vi "Create Phrase with Unit or Greek Letter.vi"(0 "Phrase IN":refnum<k24>, 2 "Exponent rise":sgl, 5 "Greek Font Ref":refnum<k24>, 7 "Exponent Font Ref":refnum<k24>, 9 "Cell Font Ref":refnum<k24>, 11 "error in (no error)":errorcluster, 13 "String":string) -> (4 "Phrase OUT reference 2":refnum<k24>, 15 "error out":errorcluster)   [LabVIEW 2019]
doc: "Appends <B>text</B> in a column header (or footer). You can use this polymorphic VI to append a colomn to a header (or footer). The data type you wire to the <B>Header or footer</B> input determines the polymorphic instance to use.\n\nThe header (or footer) can be divided up into three columns. Each column has the same width. The number of header (or footer) that you add determines the number of columns.\n\n<B>FRANÇAIS</B>\nAjoute du <B>texte</B> dans une colonne d'un en-tête (ou d'un pied de page). Vous pouvez utiliser ce VI polymorphique pour ajouter une colonne à un en-tête (ou un pied de page). Le type de variable que vous reliez au terminal <B>Header or footer</B> détermine l'instance polymorphique à utiliser.\n\nL'en-tête (ou le pied de page) peut être divisé en un maximum de trois colonnes. Chaque colonne a la même largeur. Le nombre d'en-têtes (ou de pieds de page) que vous ajoutez détermine le nombre de colonnes.\n\n\n\nVersion 1.0\nDeveloped by Jean-Marc Simard\nCopyright © 2012, Exaprom Inc.\nAll rights reserved.\nLicense: BSD\n\nWith iTextSharp 4.1.6 (http://itextsharp.sourceforge.net)\nunder Mozilla Public License Version 1.1\n(http://www.mozilla.org/MPL/MPL-1.1.html)"
uses:
  C:/Program Files/National Instruments/LabVIEW 2019/user.lib/Exaprom PDF/DLL/itextsharp.dll
  DLL/itextsharp.dll
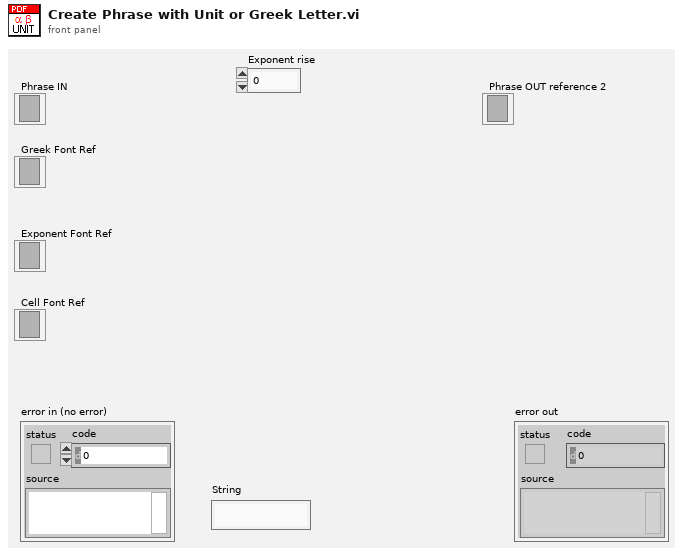
[diagram p1: front panel]
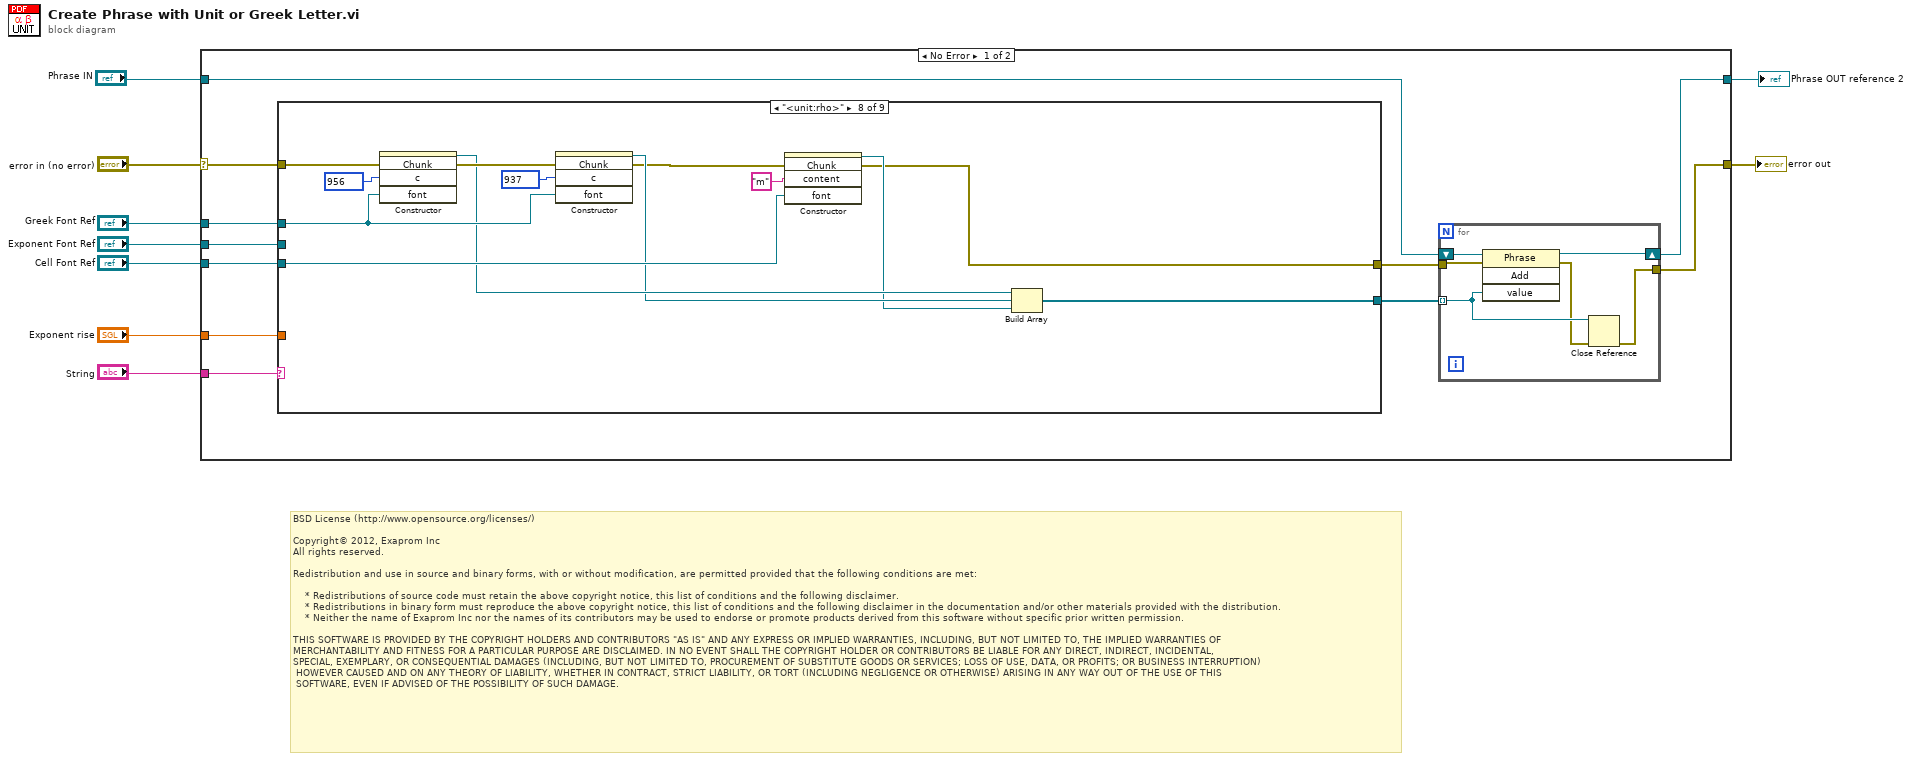
[diagram p0: block diagram]
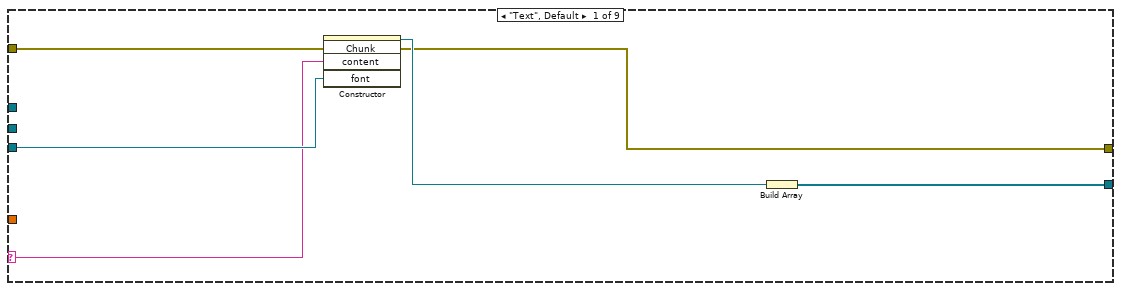
[diagram p2: hidden frame]
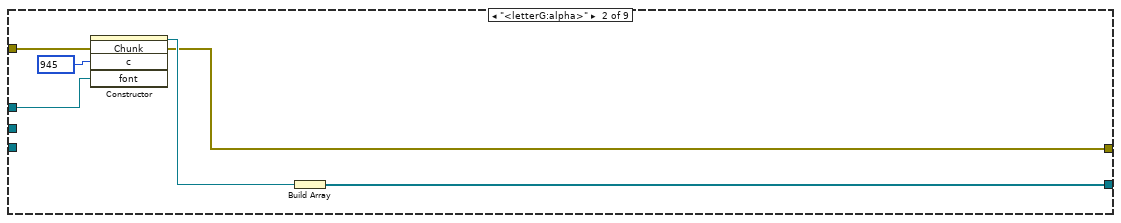
[diagram p3: hidden frame]
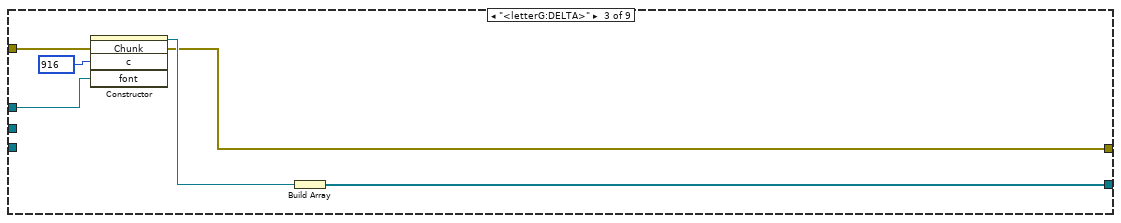
[diagram p4: hidden frame]
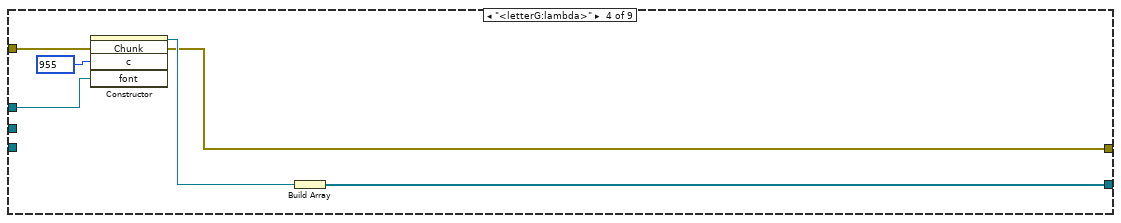
[diagram p5: hidden frame]
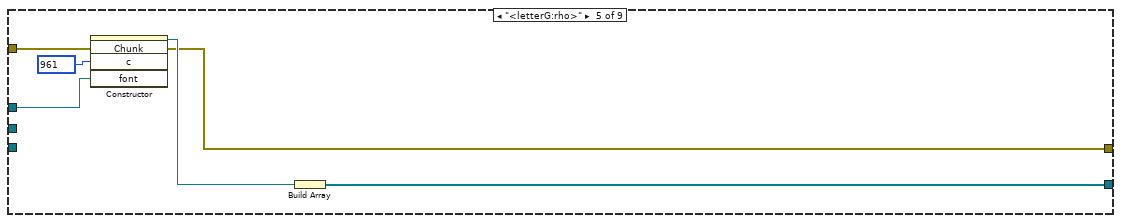
[diagram p6: hidden frame]
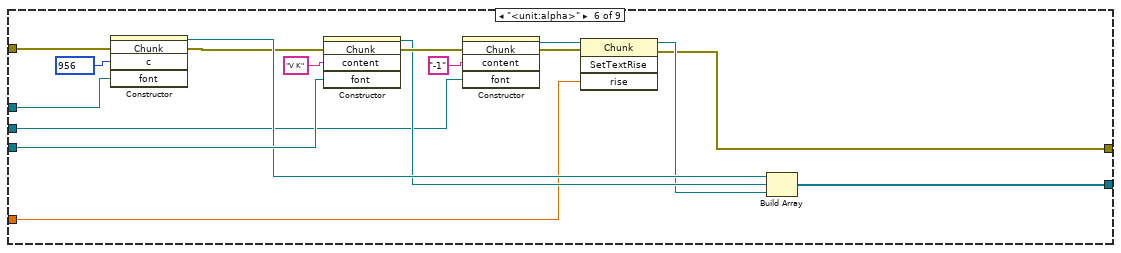
[diagram p7: hidden frame]
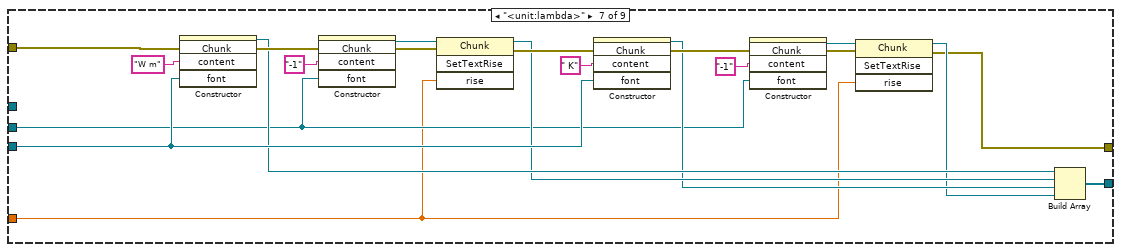
[diagram p8: hidden frame]
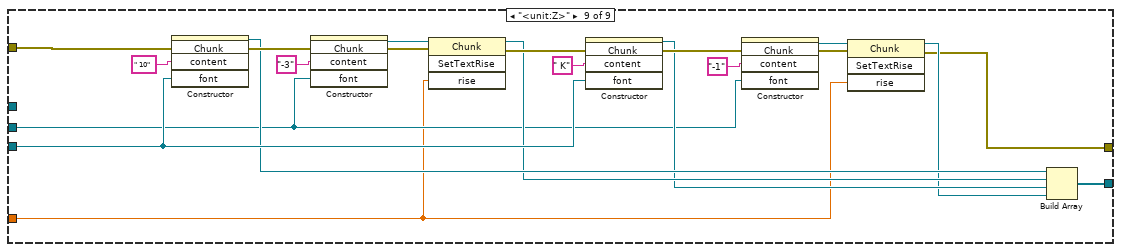
[diagram p9: hidden frame]
diagram:
  # "BSD License (http://www.opensource.org/licenses/)\n\nCopyright© 2012, Exaprom Inc\nAll rights reserved.\n\nRedistribution and use in source and binary forms, with or without modification, are permitted provided that the following conditions are met:\n\n    * Redistributions of source code must retain the above copyright notice, this list of conditions and the following disclaimer.\n    * Redistributions in binary form must reproduce the above copyright notice, this list of conditions and the following disclaimer in the documentation and/or other materials provided with the distribution.\n    * Neither the name of Exaprom Inc nor the names of its contributors may be used to endorse or promote products derived from this software without specific prior written permission.\n\nTHIS SOFTWARE IS PROVIDED BY THE COPYRIGHT HOLDERS AND CONTRIBUTORS \"AS IS\" AND ANY EXPRESS OR IMPLIED WARRANTIES, INCLUDING, BUT NOT LIMITED TO, THE IMPLIED WARRANTIES OF \nMERCHANTABILITY AND FITNESS FOR A PARTICULAR PURPOSE ARE DISCLAIMED. IN NO EVENT SHALL THE COPYRIGHT HOLDER OR CONTRIBUTORS BE LIABLE FOR ANY DIRECT, INDIRECT, INCIDENTAL,\nSPECIAL, EXEMPLARY, OR CONSEQUENTIAL DAMAGES (INCLUDING, BUT NOT LIMITED TO, PROCUREMENT OF SUBSTITUTE GOODS OR SERVICES; LOSS OF USE, DATA, OR PROFITS; OR BUSINESS INTERRUPTION)\n HOWEVER CAUSED AND ON ANY THEORY OF LIABILITY, WHETHER IN CONTRACT, STRICT LIABILITY, OR TORT (INCLUDING NEGLIGENCE OR OTHERWISE) ARISING IN ANY WAY OUT OF THE USE OF THIS\n SOFTWARE, EVEN IF ADVISED OF THE POSSIBILITY OF SUCH DAMAGE."
  n1 = case shown="No Error" "error in (no error)" {
    selector: "error in (no error)" -> [w14 w130]
    tunnel: [w18 w130] -> w9
    tunnel: "String" -> [w19 _]
    tunnel: "Cell Font Ref" -> [w17 _]
    tunnel: "Exponent Font Ref" -> [w16 _]
    tunnel: "Greek Font Ref" -> [w15 _]
    tunnel: "Exponent rise" -> [w13 _]
    tunnel: [w12 w129] -> w2
    tunnel: "Phrase IN" -> [w10 w129]
    frame No Error {
      n2 = case shown="\"<unit:rho>\"" w19 {
        selector: w19 -> [w23 _ _ _ _ _ _ _ _]
        tunnel: [w26 w28 w34 w40 w46 w65 w86 w99 w120] -> w20
        tunnel: w17 -> [w25 _ _ _ _ w60 w76 w98 w110]
        tunnel: w16 -> [_ _ _ _ _ w56 w71 _ w105]
        tunnel: [w21 w27 w33 w39 w45 w52 w68 w89 w103] -> w11
        tunnel: w13 -> [_ _ _ _ _ w55 w70 _ w104]
        tunnel: w14 -> [w22 w31 w37 w43 w49 w54 w69 w97 w102]
        tunnel: w15 -> [_ w30 w36 w42 w48 w53 _ w94 _]
        frame "Text", Default {
          n3 = constructor class="Chunk"(error in=w22, "content"=w23, "font"=w25) -> (reference out=w24:refnum<k24>, error out=w21:errorcluster)  [unwired: 2 in, 3 out]
          n4 = Build Array(w24) -> (w26:refnum<k24>[])
        }
        frame "<letterG:alpha>" {
          n5 = constructor class="Chunk"(error in=w31, "c"=u16 945, "font"=w30) -> (reference out=w29:refnum<k24>, error out=w27:errorcluster)  [unwired: 2 in, 3 out]
          n6 = Build Array(w29) -> (w28:refnum<k24>[])
        }
        frame "<letterG:DELTA>" {
          n7 = constructor class="Chunk"(error in=w37, "c"=u16 916, "font"=w36) -> (reference out=w35:refnum<k24>, error out=w33:errorcluster)  [unwired: 2 in, 3 out]
          n8 = Build Array(w35) -> (w34:refnum<k24>[])
        }
        frame "<letterG:lambda>" {
          n9 = constructor class="Chunk"(error in=w43, "c"=u16 955, "font"=w42) -> (reference out=w41:refnum<k24>, error out=w39:errorcluster)  [unwired: 2 in, 3 out]
          n10 = Build Array(w41) -> (w40:refnum<k24>[])
        }
        frame "<letterG:rho>" {
          n11 = constructor class="Chunk"(error in=w49, "c"=u16 961, "font"=w48) -> (reference out=w47:refnum<k24>, error out=w45:errorcluster)  [unwired: 2 in, 3 out]
          n12 = Build Array(w47) -> (w46:refnum<k24>[])
        }
        frame "<unit:alpha>" {
          n13 = constructor class="Chunk"(error in=w54, "c"=u16 956, "font"=w53) -> (reference out=w59:refnum<k24>, error out=w51:errorcluster)  [unwired: 2 in, 3 out]
          n14 = constructor class="Chunk"(error in=w51, "content"="V K", "font"=w60) -> (reference out=w58:refnum<k24>, error out=w61:errorcluster)  [unwired: 2 in, 3 out]
          n15 = constructor class="Chunk"(error in=w61, "content"="-1", "font"=w56) -> (reference out=w62:refnum<k24>, error out=w63:errorcluster)  [unwired: 2 in, 3 out]
          n16 = invoke class="Chunk" method="SetTextRise"(reference=w62, error in=w63, "rise"=w55) -> (reference out=w57:refnum<k24>, error out=w52:errorcluster)  [unwired: 1 in, 2 out]
          n17 = Build Array(w59, w58, w57) -> (w65:refnum<k24>[])
        }
        frame "<unit:lambda>" {
          n18 = constructor class="Chunk"(error in=w69, "content"="W m", "font"=w76) -> (reference out=w75:refnum<k24>, error out=w79:errorcluster)  [unwired: 2 in, 3 out]
          n19 = constructor class="Chunk"(error in=w79, "content"="-1", "font"=w71) -> (reference out=w80:refnum<k24>, error out=w81:errorcluster)  [unwired: 2 in, 3 out]
          n20 = invoke class="Chunk" method="SetTextRise"(reference=w80, error in=w81, "rise"=w70) -> (reference out=w74:refnum<k24>, error out=w78:errorcluster)  [unwired: 1 in, 2 out]
          n21 = constructor class="Chunk"(error in=w78, "content"=" K", "font"=w76) -> (reference out=w73:refnum<k24>, error out=w77:errorcluster)  [unwired: 2 in, 3 out]
          n22 = constructor class="Chunk"(error in=w77, "content"="-1", "font"=w71) -> (reference out=w85:refnum<k24>, error out=w84:errorcluster)  [unwired: 2 in, 3 out]
          n23 = invoke class="Chunk" method="SetTextRise"(reference=w85, error in=w84, "rise"=w70) -> (reference out=w72:refnum<k24>, error out=w68:errorcluster)  [unwired: 1 in, 2 out]
          n24 = Build Array(w75, w74, w73, w72) -> (w86:refnum<k24>[])
        }
        frame "<unit:rho>" {
          n25 = constructor class="Chunk"(error in=w97, "c"=u16 956, "font"=w94) -> (reference out=w93:refnum<k24>, error out=w95:errorcluster)  [unwired: 2 in, 3 out]
          n26 = constructor class="Chunk"(error in=w95, "c"=u16 937, "font"=w94) -> (reference out=w92:refnum<k24>, error out=w90:errorcluster)  [unwired: 2 in, 3 out]
          n27 = constructor class="Chunk"(error in=w90, "content"="m", "font"=w98) -> (reference out=w91:refnum<k24>, error out=w89:errorcluster)  [unwired: 2 in, 3 out]
          n28 = Build Array(w93, w92, w91) -> (w99:refnum<k24>[])
        }
        frame "<unit:Z>" {
          n29 = constructor class="Chunk"(error in=w102, "content"=" 10", "font"=w110) -> (reference out=w109:refnum<k24>, error out=w113:errorcluster)  [unwired: 2 in, 3 out]
          n30 = constructor class="Chunk"(error in=w113, "content"="-3", "font"=w105) -> (reference out=w114:refnum<k24>, error out=w115:errorcluster)  [unwired: 2 in, 3 out]
          n31 = invoke class="Chunk" method="SetTextRise"(reference=w114, error in=w115, "rise"=w104) -> (reference out=w108:refnum<k24>, error out=w112:errorcluster)  [unwired: 1 in, 2 out]
          n32 = constructor class="Chunk"(error in=w112, "content"=" K", "font"=w110) -> (reference out=w107:refnum<k24>, error out=w111:errorcluster)  [unwired: 2 in, 3 out]
          n33 = constructor class="Chunk"(error in=w111, "content"="-1", "font"=w105) -> (reference out=w119:refnum<k24>, error out=w118:errorcluster)  [unwired: 2 in, 3 out]
          n34 = invoke class="Chunk" method="SetTextRise"(reference=w119, error in=w118, "rise"=w104) -> (reference out=w106:refnum<k24>, error out=w103:errorcluster)  [unwired: 1 in, 2 out]
          n35 = Build Array(w109, w108, w107, w106) -> (w120:refnum<k24>[])
        }
      }
      n36 = for {
        shift-right: [w127] -> w12
        shift-left: w10 -> [w128]
        tunnel: w11 -> [w124]
        tunnel: w20 -> [w126] mode=indexing
        tunnel: [w123] -> w18
        n37 = invoke class="Phrase" method="Add"(reference=w128, error in=w124, "value"=w126) -> (reference out=w127:refnum<k24>, error out=w125:errorcluster)  [unwired: 1 in, 2 out]
        n38 = Close Reference(reference=w126, error in (no error)=w125) -> (error out=w123:errorcluster)
      }
    }
    frame Error {
    }
  }
  "error out" <- w9
  "Phrase OUT reference 2" <- w2
